vi "MEMR-Plot Mag Spectra.vi"(0 "Spectra":cluster{"Freq (Hz)":dbl[], "Mag":dbl[][]}[](array[cluster]), 1 "Spectrum":refnum<vi>, 5 "Fmax":dbl=8000.0 format="%#_13g", 7 "Fpeak":dbl[](array[numeric]), 9 "Noise floor":cluster{"Freq (Hz)":dbl[], dbl[]}[](array[cluster]), 11 "error in (no error)":errorcluster, 12 "plotWhich":i32) -> (15 "error out":errorcluster)   [LabVIEW 2020]
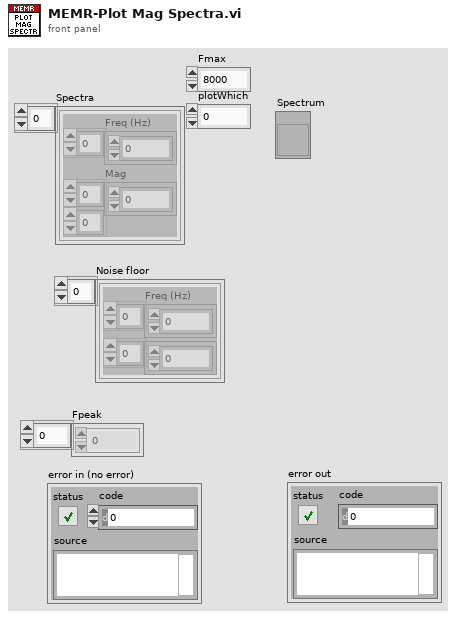
[diagram p1: front panel]
types:
  T1 = enum16{"User", "Prism", "Kelly", "Dark2", "Sequential", "Hue"}
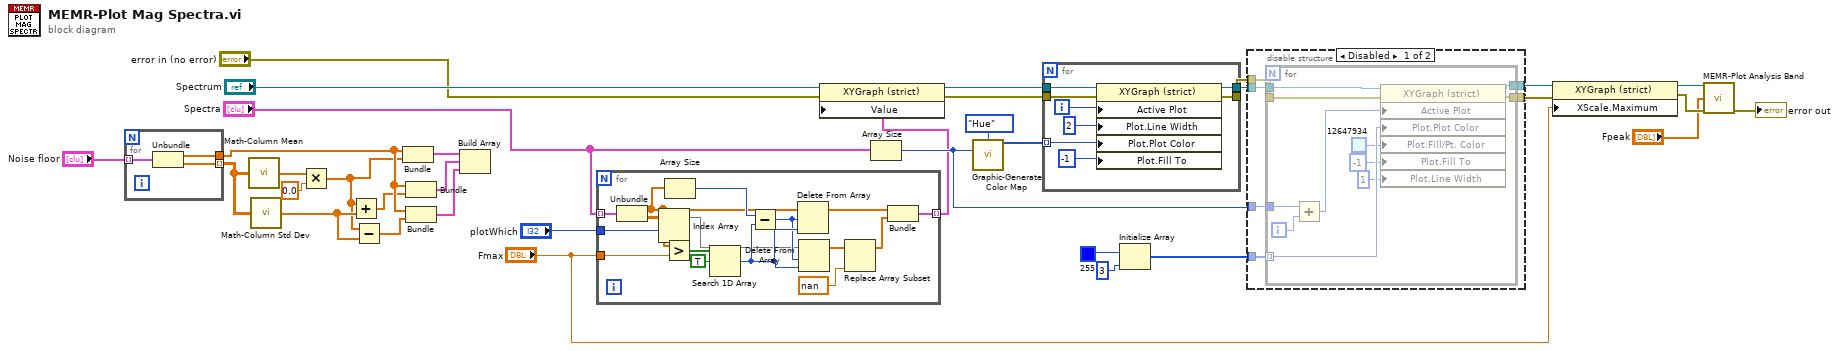
[diagram p0: block diagram]
diagram:
  n1 = for {
    tunnel: "Noise floor" -> [w37] mode=indexing
    tunnel: [w36] -> w24 mode=indexing
    tunnel: [w35] -> w25
    n2 = Unbundle(w37) -> ("Freq (Hz)"=w35:dbl[], w36:dbl[])
  }
  n3 = call "Math-Column Mean.vi"("2D Array"=w24) -> ("Column means"=w16:dbl[])
  n4 = call "Math-Column Std Dev.vi"("2D Array"=w24) -> ("Column means"=w17:dbl[])
  n5 = Multiply(x=w16, y=0.0) -> (x*y=w11:dbl[])
  n6 = Add(x=w11, y=w17) -> (x+y=w18:dbl[])
  n7 = Subtract(x=w11, y=w17) -> (x-y=w19:dbl[])
  n8 = Bundle("Freq (Hz)"=w25, w11) -> (w20:cluster{"Freq (Hz)":dbl[], dbl[]})  [unwired: 1 in]
  n9 = Bundle("Freq (Hz)"=w25, w18) -> (w21:cluster{"Freq (Hz)":dbl[], dbl[]})  [unwired: 1 in]
  n10 = Bundle("Freq (Hz)"=w25, w19) -> (w22:cluster{"Freq (Hz)":dbl[], dbl[]})  [unwired: 1 in]
  n11 = Build Array(w20, w21, w22) -> ()  [unwired: 1 out]
  n12 = for {
    tunnel: "Spectra" -> [w53] mode=indexing
    tunnel: [w48] -> w1 mode=indexing
    tunnel: "Fmax" -> [w41]
    tunnel: "plotWhich" -> [w40]
    n13 = Unbundle(w53) -> ("Freq (Hz)"=w39:dbl[], "Mag"=w50:dbl[][])
    n14 = Index Array(array=w50, index (row)=w40) -> (element=w38:dbl[])  [unwired: 1 in]
    n15 = Greater?(x=w39, y=w41) -> (0:w52:bool[])
    n16 = Array Size(array=w39) -> (size(s)=w47:i32)
    n17 = Search 1D Array(1D array=w52, element=TRUE) -> (index of element=w46:i32)  [unwired: 1 in]
    n18 = Subtract(x=w47, y=w46) -> (x-y=w45:i32)
    n19 = Delete From Array(array=w39, length=w45, index=w46) -> (array with subset deleted=w49:dbl[])  [unwired: 1 out]
    n20 = Delete From Array(array=w38, length=w45, index=w46) -> (array with subset deleted=w44:dbl[])  [unwired: 1 out]
    n21 = Replace Array Subset(array=w44, new element=nan) -> (w43:dbl[])  [unwired: 1 in]
    n22 = Bundle("Freq (Hz)"=w49, "Mag"=w43) -> (w48:cluster{"Freq (Hz)":dbl[], "Mag":dbl[]})  [unwired: 1 in]
  }
  n23 = property on="Property Node" class="XYGraph (strict)"(reference="Spectrum", error in="error in (no error)", "Value"=w1) -> (reference out=w15:refnum<vi>, error out=w32:errorcluster)
  n24 = Array Size(array="Spectra") -> (size(s)=w26:i32)
  n25 = call "Graphic-Generate Color Map.vi"("Map"=T1."Hue", "Size"=w26) -> ("Colors"=w33:u32[])  [unwired: 13 in]
  n26 = for {
    tunnel: w33 -> [w59] mode=indexing
    tunnel: w32 -> [w58]
    tunnel: [w57] -> w29
    tunnel: w15 -> [w55]
    tunnel: [w54] -> w14
    i -> [w61]
    n27 = property on="Property Node" class="XYGraph (strict)"(reference=w55, error in=w58, "Active Plot"=w61, "Plot.Line Width"=u8 2, "Plot.Plot Color"=w59, "Plot.Fill To"=i16 -1) -> (reference out=w54:refnum<vi>, error out=w57:errorcluster)
  }
  n28 = Initialize Array(u32 255, 3) -> (w28:u32[])
  n29 = disable-structure shown="Disabled" {
    disable-tunnel: w29 -> [w67 w79]
    disable-tunnel: w28 -> [w66 _]
    disable-tunnel: [w65 w79] -> w27
    disable-tunnel: w26 -> [w64 _]
    disable-tunnel: w14 -> [w63 w80]
    disable-tunnel: [w62 w80] -> w13
    frame Disabled {
      n30 = for {
        tunnel: w67 -> [w78]
        tunnel: w66 -> [w74] mode=indexing
        tunnel: w64 -> [w77]
        tunnel: [w70] -> w65
        tunnel: w63 -> [w69]
        tunnel: [w68] -> w62
        i -> [w76]
        n31 = Add(x=w77, y=w76) -> (x+y=w75:i32)
        n32 = property on="Property Node" class="XYGraph (strict)"(reference=w69, error in=w78, "Active Plot"=w75, "Plot.Plot Color"=w74, "Plot.Fill/Pt. Color"=u32 12647934, "Plot.Fill To"=i16 -1, "Plot.Line Width"=u8 1) -> (reference out=w68:refnum<vi>, error out=w70:errorcluster)
      }
    }
    frame Enabled {
    }
  }
  n33 = property on="Property Node" class="XYGraph (strict)"(reference=w13, error in=w27, "XScale.Maximum"="Fmax") -> (reference out=w7:refnum<vi>, error out=w6:errorcluster)
  n34 = call "MEMR-Plot Analysis Band.vi"("XYGraph in"=w7, "Fpeak"="Fpeak", "error in (no error)"=w6) -> ("error out"=→"error out":errorcluster)  [unwired: 12 in]
